vi "Write Test Param.vi"(8 "error in (no error)":errorcluster, 10 "Param 1":string, 11 "Test Switch Init Parameters in":refnum<class "Test Switch Init Parameters.lvclass">) -> (0 "error out":errorcluster, 3 "Test Switch Init Parameters out":refnum<class "Test Switch Init Parameters.lvclass">)   [LabVIEW 2027, in "Test Switch Init Parameters.lvclass"]
uses:
  Test Switch Init Parameters.lvclass
  Test Switch Init Parameters.lvclass/Test Switch Init Parameters.ctl
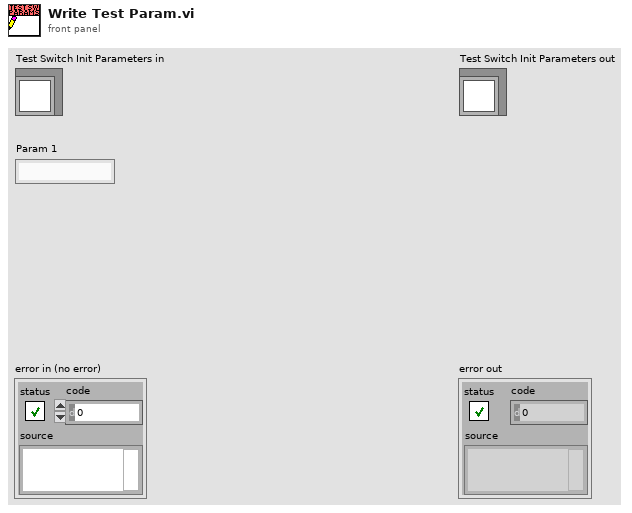
[diagram p1: front panel]
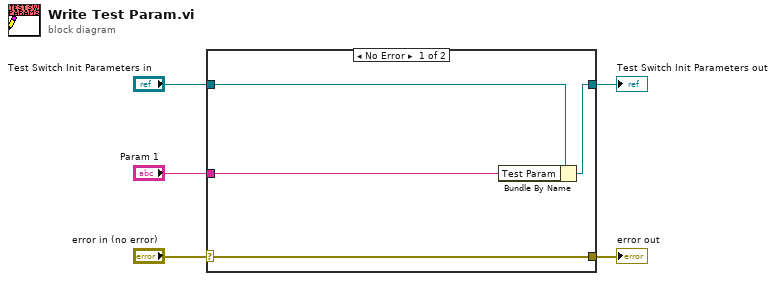
[diagram p0: block diagram]
diagram:
  n1 = case shown="No Error" "error in (no error)" {
    selector: "error in (no error)" -> [w9 w10]
    tunnel: [w9 w10] -> w4
    tunnel: [w7 w11] -> w2
    tunnel: "Test Switch Init Parameters in" -> [w8 w11]
    tunnel: "Param 1" -> [w6 _]
    frame No Error {
      n2 = Bundle By Name(cluster=w8, "Test Param"=w6) -> (w7:refnum<class "Test Switch Init Parameters.lvclass">)
    }
    frame Error {
    }
  }
  "error out" <- w4
  "Test Switch Init Parameters out" <- w2
